vi "setTCPConfiguration.vi"(8 "error in (no error)":errorcluster, 10 "Settings":T1={"IP"="127.0.0.1", "port_low"=50000, "port_up"=50000, "connection_timeout "=10, "reading_timeout"=10, "writing_timeout"=10}, 11 "tcpDevice in":refnum<class "tcpDevice.lvclass">) -> (0 "error out":errorcluster, 3 "tcpDevice out":refnum<class "tcpDevice.lvclass">)   [LabVIEW 2016, in "tcpDevice.lvclass"]
uses:
  tcpDevice.lvclass
  ts_labview_tcp/tcpTypedefs/TCPSettings.ctl
  ts_labview_tcp/TCPSettings/TCPSettings.lvclass
  ts_labview_tcp/TCPComEvents/TCPComEvents.lvclass
  tcpDevice.lvclass/tcpDevice.ctl
  ts_labview_tcp/TCPCommunicator/TCPCommunicator.lvclass/TCPCommunicator.ctl
  ts_labview_tcp/TCPClient/TCPClient.lvclass
  C:/Users/aanania/Documents/common_labview_tcpdevice/ts_labview_tcp/TCPCommunicator/TCPCommunicator.lvclass
  ts_labview_tcp/TCPCommunicator/TCPCommunicator.lvclass
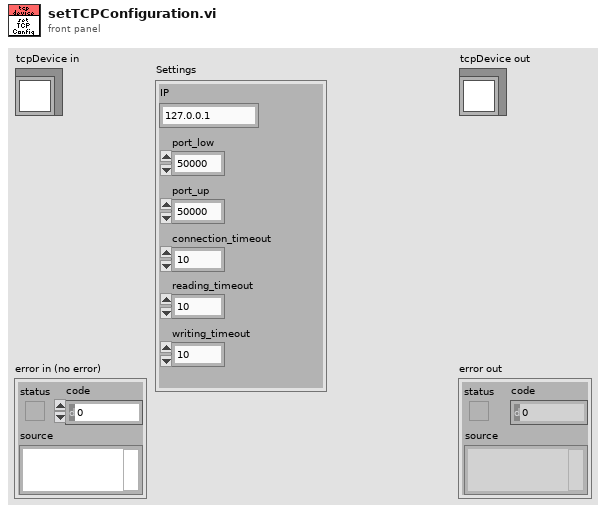
[diagram p1: front panel]
types:
  T1 = typedef "TCPSettings.ctl" = cluster{"IP":string, "port_low":u16, "port_up":u16, "connection_timeout ":i32, "reading_timeout":i32, "writing_timeout":i32}
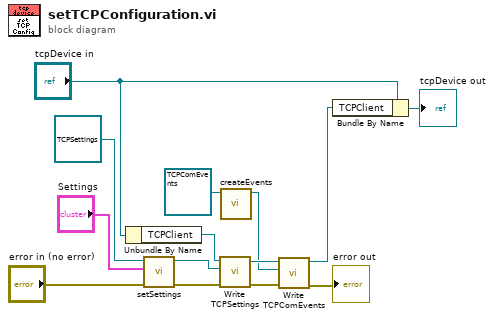
[diagram p0: block diagram]
diagram:
  n1 = Unbundle By Name("tcpDevice in") -> ("TCPClient"=w12:refnum<class "TCPClient.lvclass">)
  n2 = call "setSettings.vi"("error in (no error)"="error in (no error)", "Settings"="Settings", "TCPSettings in"=refnum<class "TCPSettings.lvclass"> refnum) -> ("error out"=w8:errorcluster, "TCPSettings out"=w7:refnum<class "TCPSettings.lvclass">)  [unwired: 7 in]
  n3 = call-dynamic "Write TCPSettings.vi"("error in (no error)"=w8, "TCPSettings.lvclass"=w7, "TCPCommunicator in"=w12) -> ("error out"=w6:errorcluster, "TCPCommunicator out"=w5:refnum<class "TCPClient.lvclass">)  [unwired: 7 in]
  n4 = call "createEvents.vi"("TCPComEvents in"=refnum<class "TCPComEvents.lvclass"> refnum) -> ("TCPComEvents out"=w1:refnum<class "TCPComEvents.lvclass">)  [unwired: 9 in, 1 out]
  n5 = call "Write TCPComEvents.vi"("error in (no error)"=w6, "TCPComEvents.lvclass"=w1, "TCPCommunicator in"=w5) -> ("error out"=→"error out":errorcluster, "TCPCommunicator out"=w4:refnum<class "TCPClient.lvclass">)  [unwired: 7 in]
  n6 = Bundle By Name(cluster="tcpDevice in", "TCPClient"=w4) -> (→"tcpDevice out":refnum<class "tcpDevice.lvclass">)
